vi "Convert to TDMS.vi"() -> ()   [LabVIEW 2019]
panel:
  out "Filename Out":path
  out "Numeric":i32
  out "Signals 2":dynamicdata(graph) caption="Signals"
  in  "In":path=path "test.lvm" caption="Filename"
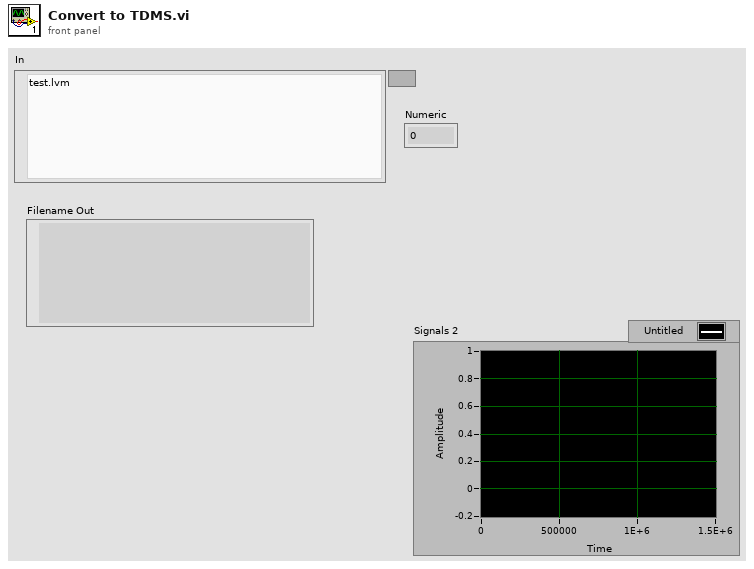
[diagram p1: front panel]
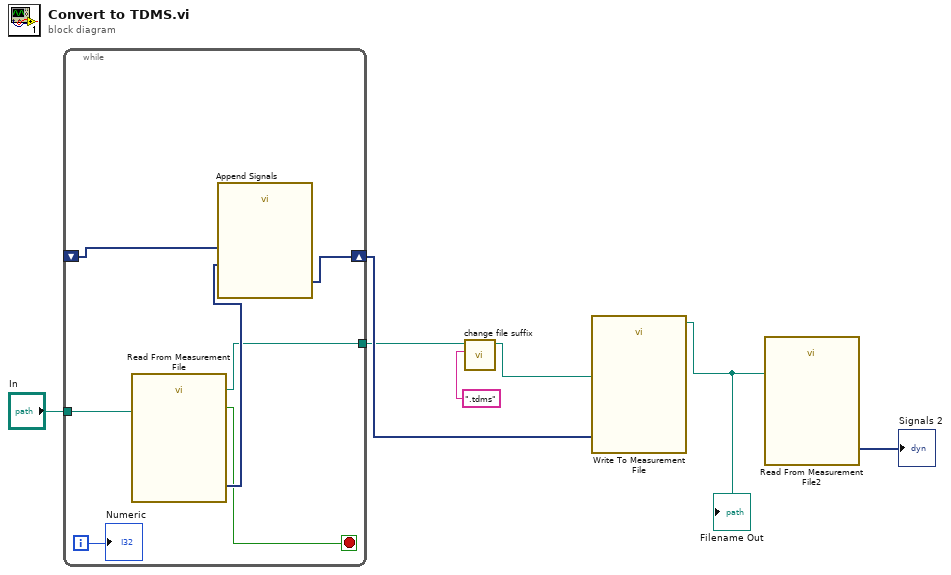
[diagram p0: block diagram]
diagram:
  n1 = while {
    shift-right: [w13] -> w5
    shift-left: _ -> [w14]
    tunnel: "In" -> [w10]
    tunnel: [w8] -> w3
    i -> [w9]
    stop <- w11 stop-if-true
    n2 = call "Read From Measurement File"("Filename"=w10) -> ("Filename Out"=w8:path, "Signals"=w12:dynamicdata, "EOF?"=w11:bool)  [unwired: 5 in, 3 out]
    n3 = call "Append Signals"("Input Signal B"=w12, "Input Signal A"=w14) -> ("Appended Signals"=w13:dynamicdata)  [unwired: 8 in, 1 out]
    "Numeric" <- w9
  }
  n4 = call "change file suffix.vi"("new suffix"=".tdms", "path"=w3) -> ("path 2"=w1:path)  [unwired: 9 in]
  n5 = call "Write To Measurement File"("Signals"=w5, "Filename"=w1) -> ("Filename Out"=w7:path)  [unwired: 15 in, 2 out]
  "Filename Out" <- w7
  n6 = call "Read From Measurement File2"("Filename"=w7) -> ("Signals"=→"Signals 2":dynamicdata)  [unwired: 5 in, 5 out]
